vi "Set Frame Transfer.vi"(8 "error in (no error)":errorcluster, 11 "CCDCamera in":refnum<class "iKon-L.lvclass">) -> (0 "error out":errorcluster, 3 "CCDCamera out":refnum<class "iKon-L.lvclass">)   [LabVIEW 2018, in "iKon-L.lvclass"]
doc: "Turn the frame trasnfer mode on or off"
uses:
  iKon-L.lvclass
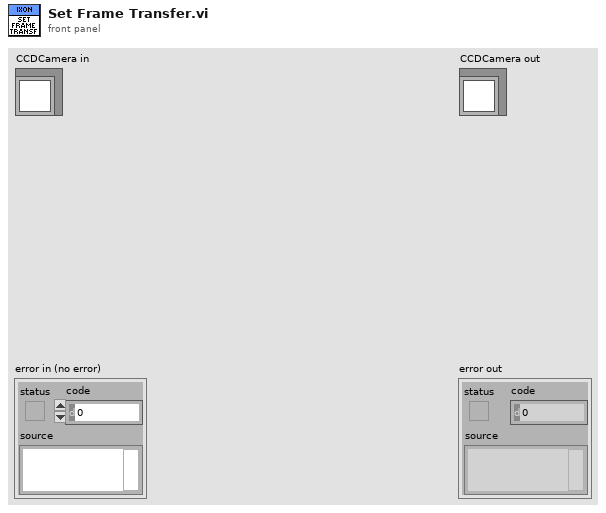
[diagram p1: front panel]
types:
  T1 = cluster{"EM_MODE":u16, "EM_GAIN":u16, "FRAME_TRANSFER":bool}
  T2 = cluster{"PREAMP":u16, "READOUT_RATE":u16, "VERTICAL_SHIFT_SPEED":u16, "READ_MODE":u16, "VERTICAL_CLOCK_VOLTAGE":u16, "ACQUISITION_MODE":u16, "AD_CHANNEL":u16, "SHUTTER_TTL":u16, "SHUTTER_OPENING_TIME":u16, "SHUTTER_CLOSING_TIME":u16, "SHUTTER_MODE":u16, "TRIGGER_MODE":u16, "VBIN":u16, "INITIAL_LINE":u16, "INITIAL_COLUMN":u16, "FINAL_LINE":u16, "FINAL_COLUMN":u16, "HBIN":u16}
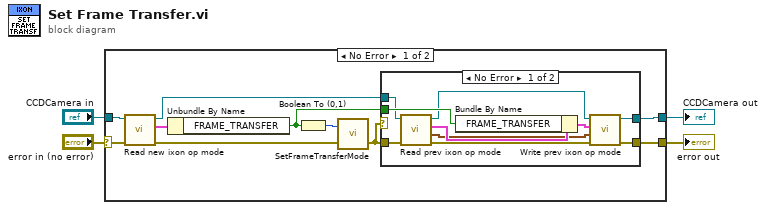
[diagram p0: block diagram]
diagram:
  n1 = case shown="No Error" "error in (no error)" {
    selector: "error in (no error)" -> [w10 w28]
    tunnel: [w13 w28] -> w4
    tunnel: [w5 w27] -> w3
    tunnel: "CCDCamera in" -> [w9 w27]
    frame No Error {
      n2 = call-dynamic "Read new ixon op mode.vi"("error in (no error)"=w10, "Sim_Ixon_Ultra in"=w9) -> ("error out"=w8:errorcluster, "new ixon op mode"=w11:T1, "Sim_Ixon_Ultra out"=w6:refnum<class "iKon-L.lvclass">)  [unwired: 6 in, 1 out]
      n3 = Unbundle By Name(w11) -> ("FRAME_TRANSFER"=w7:bool)
      n4 = Boolean To (0,1)(Boolean=w7) -> (0, 1=w14:i16)
      n5 = call <userlib>:"SetFrameTransferMode.vi"("error in (no error)"=w8, "mode"=w14) -> ("error out"=w12:errorcluster)  [unwired: 1 out]
      n6 = case shown="No Error" w12 {
        tunnel: [w18 w26] -> w13
        tunnel: w12 -> [w22 w26]
        tunnel: w7 -> [w23 _]
        tunnel: w6 -> [w21 w25]
        tunnel: [w19 w25] -> w5
        frame No Error {
          n7 = call-dynamic "Read prev ixon op mode.vi"("error in (no error)"=w22, "Sim_Ixon_Ultra in"=w21) -> ("error out"=w17:errorcluster, "prev operation mode"=w15:T2, "prev ixon op mode"=w24:T1, "Sim_Ixon_Ultra out"=w20:refnum<class "iKon-L.lvclass">)  [unwired: 6 in]
          n8 = Bundle By Name(cluster=w24, "FRAME_TRANSFER"=w23) -> (w16:T1)
          n9 = call-dynamic "Write prev ixon op mode.vi"("error in (no error)"=w17, "prev operation mode"=w15, "prev ixon op mode"=w16, "Sim_Ixon_Ultra in"=w20) -> ("error out"=w18:errorcluster, "Sim_Ixon_Ultra out"=w19:refnum<class "iKon-L.lvclass">)  [unwired: 6 in]
        }
        frame Error {
        }
      }
    }
    frame Error {
    }
  }
  "error out" <- w4
  "CCDCamera out" <- w3
